vi "Robot Values.vi"() -> ()   [LabVIEW 2014]
uses:
  <vilib>/Rock Robotics/WPI/Relay/WPI_RelayValue.ctl
panel:
  out "Auton":cluster{"Auton":string}
  in  "Tote Stopper Motors":cluster{"RelayValue":T1, "RelayValue 2":T1}
  in  "Lights":T2
  out "Lift System":T3
  out "Sensors":T4
  out "Joystick":T5
  out "Drive":T6
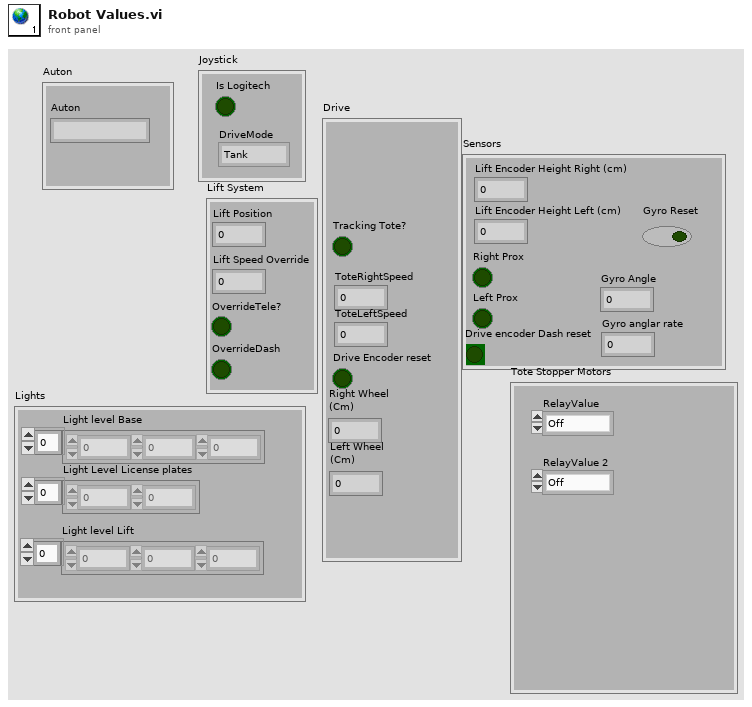
[diagram p1: front panel]
types:
  T1 = typedef "WPI_RelayValue.ctl" = enum16{"Off", "On", "Forward", "Reverse"}
  T2 = cluster{"Light level Base":dbl[], "Light level Lift":dbl[], "Light Level License plates":dbl[]}
  T3 = cluster{"Lift Position":i32, "Lift Speed Override":dbl, "OverrideTele?":bool, "OverrideDash":bool}
  T4 = cluster{"Lift Encoder Height Right (cm)":dbl, "Lift Encoder Height Left (cm)":dbl, "Right Prox":bool, "Left Prox":bool, "Gyro Angle":dbl, "Gyro anglar rate":dbl, "Gyro Reset":bool, "Drive encoder Dash reset":bool}
  T5 = cluster{"DriveMode":enum16{"Tank", "Arcade"}, "Is Logitech":bool}
  T6 = cluster{"Tracking Tote?":bool, "ToteRightSpeed":dbl, "ToteLeftSpeed":dbl, "Drive Encoder reset":bool, "Right Wheel \n(Cm)":dbl, "Left Wheel \n(Cm)":dbl}
diagram:
